vi "Exponent(SubVI).vi"(3 "Multiplier":T1, 4 "2° Digit":T2 caption="Digit", 5 "1° Digit":T2 caption="Digit") -> (1 "x*y":dbl format="%#_6f")   [LabVIEW 2018]
uses:
  Digit.ctl
  Multiplier.ctl
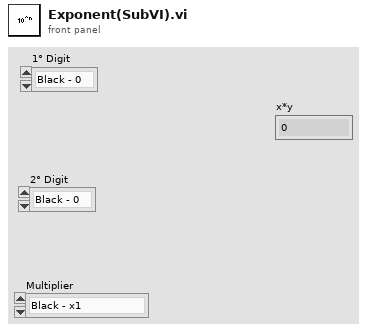
[diagram p1: front panel]
types:
  T1 = typedef "Multiplier.ctl" = enum16{"Black - x1", "Brown - x10", "Red - x100", "Orange - x1.000", "Yellow - x10.000", "Green - x100.000", "Blue - x1.000.000", "Violet -  x 10.000.000", "Grey - x100.000.000", "White - x1.000.000.000", "Silver x - 0,01", "Gold x - 0,1"}
  T2 = typedef "Digit.ctl" = enum16{"Black - 0", "Brown - 1", "Red - 2", "Orange - 3", "Yellow - 4", "Green - 5", "Blue - 6", "Violet - 7", "Grey - 8", "White - 9"}
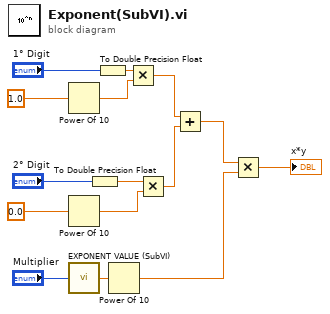
[diagram p0: block diagram]
diagram:
  n1 = Power Of 10(x=1.0) -> (10^x=w2:dbl)
  n2 = Power Of 10(x=0.0) -> (10^x=w1:dbl)
  n3 = call "EXPONENT VALUE (SubVI).vi"("Multiplier"="Multiplier") -> ("Exponent"=w3:dbl)  [unwired: 4 in]
  n4 = To Double Precision Float(number="2° Digit") -> (double precision float=w12:dbl)
  n5 = To Double Precision Float(number="1° Digit") -> (double precision float=w10:dbl)
  n6 = Power Of 10(x=w3) -> (10^x=w8:dbl)
  n7 = Multiply(x=w10, y=w2) -> (x*y=w6:dbl)
  n8 = Multiply(x=w12, y=w1) -> (x*y=w5:dbl)
  n9 = Add(x=w6, y=w5) -> (x+y=w4:dbl)
  n10 = Multiply(x=w4, y=w8) -> (x*y=→"x*y":dbl)
